vi "DM Clear.vi"(8 "error in (no error)":errorcluster) -> (0 "error out":errorcluster)   [LabVIEW 2019, in "DataManagment.lvlib"]
uses:
  DataManagment.lvlib
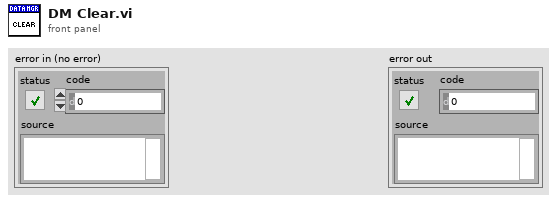
[diagram p1: front panel]
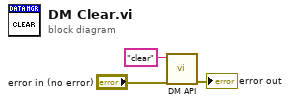
[diagram p0: block diagram]
diagram:
  n1 = call "DM API.vi"("error in (no error)"="error in (no error)", "message"="clear") -> ("error out"=→"error out":errorcluster)  [unwired: 6 in, 3 out]
